vi "ZeroGenerator.vi"(6 "Type":string(combo), 8 "Intensities":dbl[](array[numeric]), 11 "Wavelengths":dbl[](array[numeric])) -> (3 "Zero fit":dbl[](array[numeric]))   [LabVIEW 2014]
uses:
  <vilib>/Analysis/NI_AALPro.lvlib
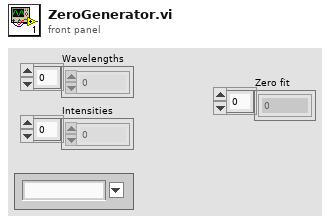
[diagram p1: front panel]
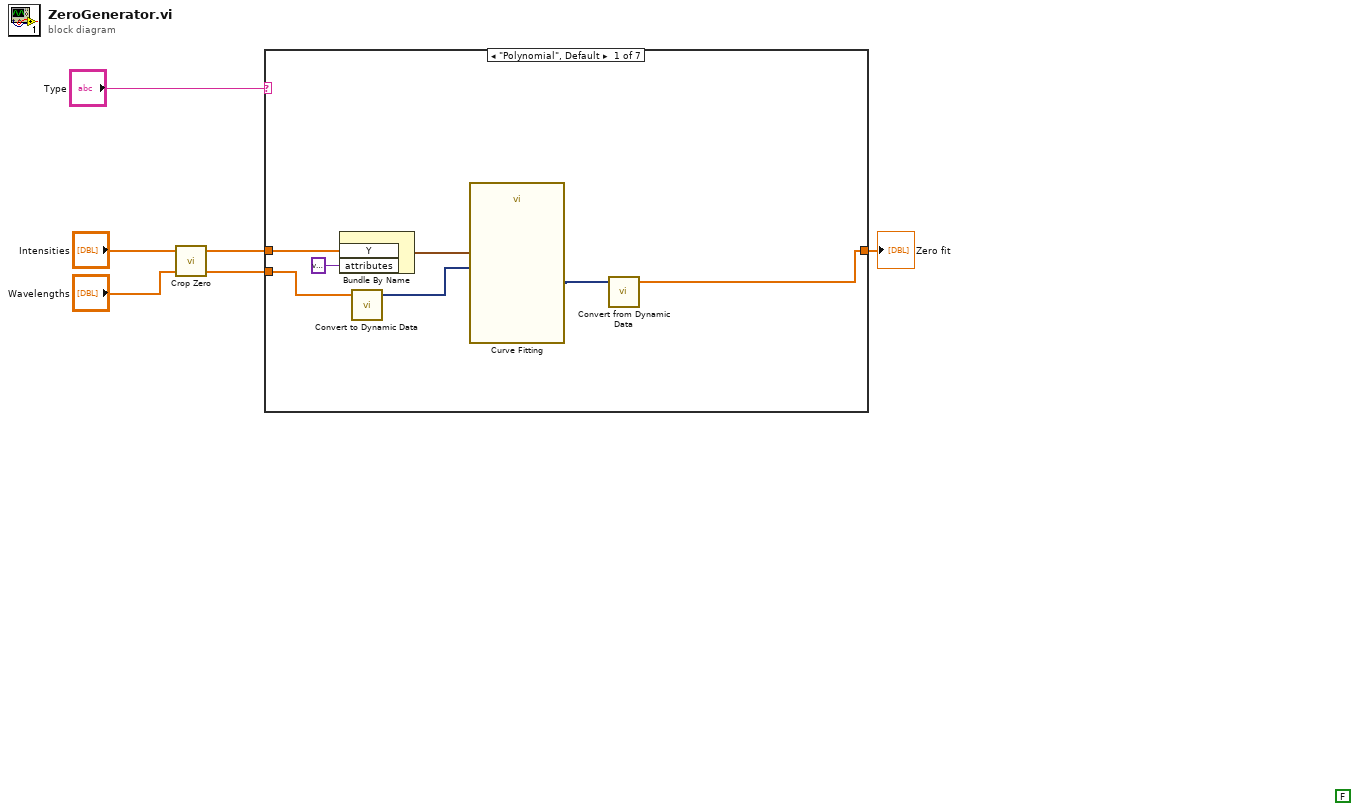
[diagram p0: block diagram]
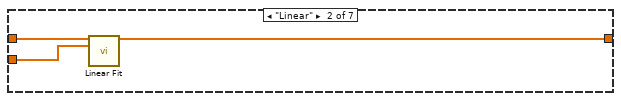
[diagram p2: hidden frame]
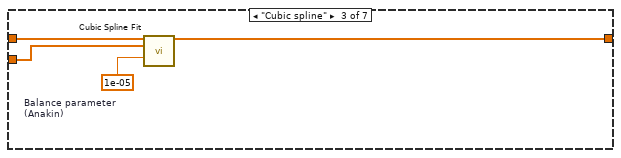
[diagram p3: hidden frame]
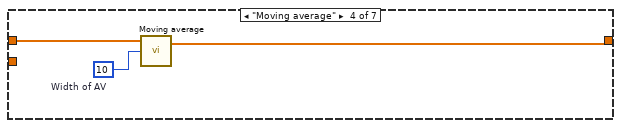
[diagram p4: hidden frame]
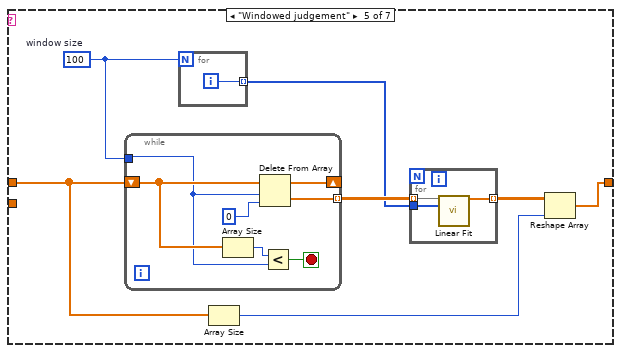
[diagram p5: hidden frame]
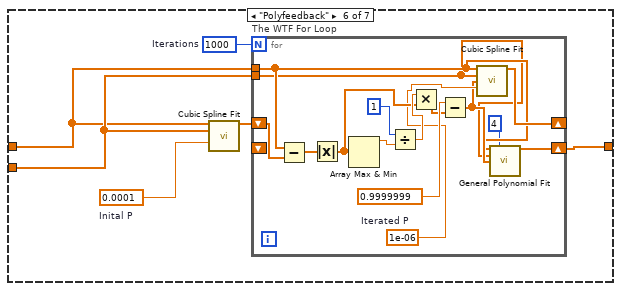
[diagram p6: hidden frame]
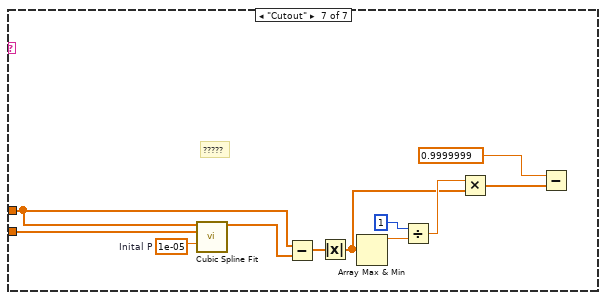
[diagram p7: hidden frame]
diagram:
  (unwired) FALSE
  n1 = call "Crop Zero.vi"("Search data"="Wavelengths", "Paired data"="Intensities") -> ("Searched data out"=w2:dbl[], "Paired data out"=w5:dbl[])  [unwired: 2 in]
  n2 = case shown="\"Polynomial\", Default" "Type" {
    tunnel: w5 -> [w10 w16 w19 w23 w27 w42 w66]
    tunnel: w2 -> [w9 w15 w18 _ _ w45 w73]
    tunnel: [w7 w14 w20 w21 w28 w43 _] -> w1
    frame "Polynomial", Default {
      n3 = Bundle By Name("Y"=w10, "attributes"=variant) -> (w13:waveform(dbl))  [unwired: 1 in]
      n4 = call "Convert to Dynamic Data"("Array"=w9) -> ("Dynamic Data Type"=w12:dynamicdata)  [unwired: 3 in]
      n5 = call "Curve Fitting"("Locations"=w12, "Signals"=w13) -> ("best fit"=w8:dynamicdata)  [unwired: 5 in, 4 out]
      n6 = call "Convert from Dynamic Data"("Dynamic Data Type"=w8) -> ("Array"=w7:dbl[])  [unwired: 3 in]
    }
    frame "Linear" {
      n7 = call <vilib>:"Linear Fit.vi"("Y"=w16, "X"=w15) -> ("Best Linear Fit"=w14:dbl[])  [unwired: 9 in, 4 out]
    }
    frame "Cubic spline" {
      w17 = 1e-05  # Balance parameter  (Anakin)
      n8 = call <vilib>:"Cubic Spline Fit.vi"("Y"=w19, "X"=w18, "balance parameter"=w17) -> ("Best Cubic Spline Fit"=w20:dbl[])  [unwired: 11 in, 1 out]
    }
    frame "Moving average" {
      w22 = 10  # Width of AV
      n9 = call "Moving average.vi"("Width of AV"=w22, "Raw data"=w23) -> ("Data AVs"=w21:dbl[])  [unwired: 1 in, 1 out]
    }
    frame "Windowed judgement" {
      w25 = 100  # window size
      n10 = while {
        tunnel: w25 -> [w36]
        shift-right: [w40] -> _
        shift-left: w27 -> [w38]
        tunnel: [w39] -> w30 mode=indexing
        stop <- w35 stop-if-true
        n11 = Array Size(array=w38) -> (size(s)=w37:i32)
        n12 = Delete From Array(array=w38, length=w36, index=0) -> (deleted portion=w39:dbl[], array with subset deleted=w40:dbl[])
        n13 = Less?(x=w37, y=w36) -> (x < y?=w35:bool)
      }
      n14 = for {
        N: w25 -> [_]
        tunnel: [w31] -> w24 mode=indexing
        i -> [w31]
      }
      n15 = Array Size(array=w27) -> (size(s)=w26:i32)
      n16 = for {
        tunnel: w30 -> [w34] mode=indexing
        tunnel: [w33] -> w29 mode=indexing
        tunnel: w24 -> [w32]
        n17 = call <vilib>:"Linear Fit.vi"("Y"=w34, "X"=w32) -> ("Best Linear Fit"=w33:dbl[])  [unwired: 9 in, 4 out]
      }
      n18 = Reshape Array(w29, w26) -> (w28:dbl[])
    }
    frame "Polyfeedback" {
      w47 = 0.0001  # Inital P
      w44 = 1000  # Iterations
      n19 = call <vilib>:"Cubic Spline Fit.vi"("Y"=w42, "X"=w45, "balance parameter"=w47) -> ("Best Cubic Spline Fit"=w46:dbl[])  [unwired: 11 in, 1 out]
      n20 = for "The WTF For Loop" {
        N: w44 -> [_]
        tunnel: w42 -> [w51]
        tunnel: w45 -> [w50]
        shift-right: [w54] -> _
        shift-left: w46 -> [w59]
        shift-right: [w48] -> w43
        shift-left: _ -> [_]
        w53 = 1e-06  # Iterated P
        n21 = Subtract(x=w51, y=w59) -> (x-y=w58:dbl[])
        n22 = Absolute Value(x=w58) -> (abs(x)=w57:dbl[])
        n23 = Array Max & Min(array=w57) -> (max value=w62:dbl)  [unwired: 3 out]
        n24 = Divide(x=1, y=w62) -> (x/y=w60:dbl)
        n25 = Multiply(x=w60, y=w57) -> (x*y=w55:dbl[])
        n26 = Subtract(x=0.9999999, y=w55) -> (x-y=w52:dbl[])
        n27 = call <vilib>:"Cubic Spline Fit.vi"("Y"=w51, "X"=w50, "Weight"=w52, "balance parameter"=w53) -> ("Best Cubic Spline Fit"=w54:dbl[])  [unwired: 10 in, 1 out]
        n28 = call <vilib>:"General Polynomial Fit.vi"("Y"=w51, "polynomial order"=4, "X"=w50, "Weight"=w52) -> ("Best Polynomial Fit"=w48:dbl[])  [unwired: 8 in, 3 out]
      }
    }
    frame "Cutout" {
      w72 = 1e-05  # Inital P
      # "?????"
      n29 = call <vilib>:"Cubic Spline Fit.vi"("Y"=w66, "X"=w73, "balance parameter"=w72) -> ("Best Cubic Spline Fit"=w63:dbl[])  [unwired: 11 in, 1 out]
      n30 = Subtract(x=w66, y=w63) -> (x-y=w68:dbl[])
      n31 = Absolute Value(x=w68) -> (abs(x)=w67:dbl[])
      n32 = Array Max & Min(array=w67) -> (max value=w71:dbl)  [unwired: 3 out]
      n33 = Divide(x=1, y=w71) -> (x/y=w69:dbl)
      n34 = Multiply(x=w69, y=w67) -> (x*y=w65:dbl[])
      n35 = Subtract(x=0.9999999, y=w65) -> ()  [unwired: 1 out]
    }
  }
  "Zero fit" <- w1
